vi "FPGA_Main_triple_SCTL.vi"() -> ()   [LabVIEW 2018]
uses:
  param-sctl-pll.ctl
  param-sctl-lockin.ctl
  scan param.ctl
  shutter-modes.ctl
  states.ctl
  <vilib>/Platform/TimedLoop/XDataNode/timing_clust.ctl
  <vilib>/Platform/TimedLoop/XDataNode/nitl_modes.ctl
  <vilib>/Platform/TimedLoop/XDataNode/wakeup.ctl
  <vilib>/rvi/Emulation/niFpgaGetClockAttributes.vi
  <vilib>/rvi/Emulation/niFpgaSctlEmulationGetInTimedLoop.vi
  <vilib>/rvi/Emulation/niFpgaEmulationReportErrorSimple.vi
  <vilib>/rvi/eio/common/nirviEmuTemplatePropertySet_noerrors.vi
  <vilib>/rvi/Emulation/niFpgaCriticalErrorInLSC.vi
  <vilib>/rvi/Emulation/niFpgaEmulationIsFPGAContextNoSignature.vi
  <vilib>/rvi/errors/niFpgaSetErrorForExecOnDevCompSimple.vi
  <vilib>/rvi/eio/common/nirviEmuReportErrorAndStop.vi
  <vilib>/rvi/DataTransferAndStorage/Container/Common/niFpgaContainerGetUniqueNameForEmu.vi
  <vilib>/rvi/FIFO/Fifo_Resource/nirvififoEmulationSetSize.vi
  <vilib>/rvi/FIFO/Fifo_Resource/nirviFifoEmulationQueueMgr.vi
  <instcachedir>/0/nirviFifoEmulationQueueMgr_E5CAEC123FF24DC58D834DCA3CDAA9B5.lvgen/nirviFifoEmulationQueueMgr_E5CAEC123FF24DC58D834DCA3CDAA9B5_000.vi
  <vilib>/Utility/error.llb/Clear Errors.vi
  <vilib>/rvi/FIFO/Fifo_Resource/nirvififoEmulationCreateLock.vi
  <vilib>/rvi/Emulation/niFpgaProcessEmulError.vi
  <vilib>/rvi/FIFO/Fifo_Resource/nirvififoEmulationObtainLock.vi
  <vilib>/rvi/FIFO/Fifo_Resource/nirvififoEmulationReleaseLock.vi
  <vilib>/rvi/occurrence/nirviWaitOnOccurrenceBase.vi
  <vilib>/rvi/errors/nirviReportUnexpectedCaseInternalError.vi
  <vilib>/rvi/errors/nirviReportUnexpectedCaseInternalError (U32).vi
  <vilib>/rvi/interface/RandomDataEmulation/niFpgaRandomDataHandleErrors.vi
  <vilib>/rvi/eio/common/nirviEmuTemplateMethod_errors.vi
  <vilib>/eio/EIOPropertyNode/EIOPropertyNode.xnode
  <vilib>/rvi/DataTransferAndStorage/Container/XNode/niFpgaContainer.xnode
  <vilib>/rvi/FIFO/Fifo_Resource/nirvififoEmulationRead.vi
  <vilib>/rvi/interface/RandomDataEmulation/nirviRandomDataFpgaReadWriteTemplate.vi
  <vilib>/eio/EIONode/EIONode.xnode
  <vilib>/Platform/TimedLoop/XDataNode/XDataNode.xnode
  <vilib>/rvi/DataTransferAndStorage/Handshake/Emulation/niFpgaHandshakeEmulation.vi
  <vilib>/rvi/eio/common/nirviEmuTemplatePropertyGet_errors.vi
  <vilib>/rvi/eio/common/nirviEmuTemplatePropertyGet_noerrors.vi
  <vilib>/rvi/eio/common/nirviEmuTemplatePropertySet_errors.vi
  PLL.lvlib
  SCTL.lvlib
  <vilib>/Platform/TimedLoop/XDataNode/XDNodeRunTimeDep.lvlib
  trigger-out.lvlib
  state machine.lvlib
panel:
  in  "enable BG log":bool
  out "APDs 2":u32[](array[numeric])
  out "x-y":u32[](array[numeric])
  out "APDs":u32[](array[numeric])
  in  "states":T1
  in  "stop":bool
  out "APDs pre-pixel":u32[](array[numeric])
  out "pixel counter":i16
  in  "line go!":bool
  out "curr state":T1
  in  "scan param":T2 {"pixel integration time (us)" format="%.2p"; "wait smaract (us)" format="%.2p"}
  out "Diode-in":fxp<+/-,27,5>
  in  "decimate":u8=1
  in  "analogue in settings":T4={"gain ch1"=1.0, "Voltage Range ch1"=enum."+/- 10 V", "gain ch2"=1.0, "Voltage Range ch1 2"=enum."+/- 10 V"}
  out "magnitude out":fxp<+,16,1>[](array[numeric])
  out "phases out":fxp<+,26,12>[](array[numeric])
  in  "param Lockin":T5={"harmonic"=[63.99993896484375, 63.99993896484375, 63.99993896484375], "LP1 coeffs"=[-1025014616, 2098093632, 165702, -1053286467, 2126356551, 167935, -1025014616, 2098093632, 165702, -1053286467, 2126356551, 167935, -1025014616, 2098093632, 165702, -1053286467, 2126356551, 167935], "scope on"=FALSE, "scope channel"=0, "scope signal"=0}
  in  "param PLL2":T6={"base freq (Hz)"=[20123.0, 20123.0, 20123.0], "P gain"=[1234.0, 1234.0, 1234.0], "I gain"=[1.0, 1.0, 1.0], "LP1 coeffs"=[-1025014616, 2098093632, 165702, -1053286467, 2126356551, 167935, -1025014616, 2098093632, 165702, -1053286467, 2126356551, 167935, -1025014616, 2098093632, 165702, -1053286467, 2126356551, 167935], "scope on"=FALSE, "scope channel"=0, "scope signal"=0, "notch coeff"=[-1025014616, 2098093632, 165702, -1053286467, 2126356551, 167935, -1025014616, 2098093632, 165702]}
  in  "param PLL1":T6={"base freq (Hz)"=[20123.0, 20123.0, 20123.0], "P gain"=[1234.0, 1234.0, 1234.0], "I gain"=[1.0, 1.0, 1.0], "LP1 coeffs"=[-1025014616, 2098093632, 165702, -1053286467, 2126356551, 167935, -1025014616, 2098093632, 165702, -1053286467, 2126356551, 167935, -1025014616, 2098093632, 165702, -1053286467, 2126356551, 167935], "scope on"=FALSE, "scope channel"=0, "scope signal"=0, "notch coeff"=[-1025014616, 2098093632, 165702, -1053286467, 2126356551, 167935, -1025014616, 2098093632, 165702]}
  out "phase error mean":fxp<+,16,1>[](array[numeric])
  out "freq error mean":fxp<+/-,16,11>[](array[numeric])
  in  "reset 3":bool
  out "AI data send at step #":i32=43
  in  "wait (clk)":u32=2 caption="wait"
  in  "idx  chan":u8
  out "timing wrong!":bool=TRUE
  out "loop time":u32=40
  in  "idx scope":u8=1
  in  "reset":bool
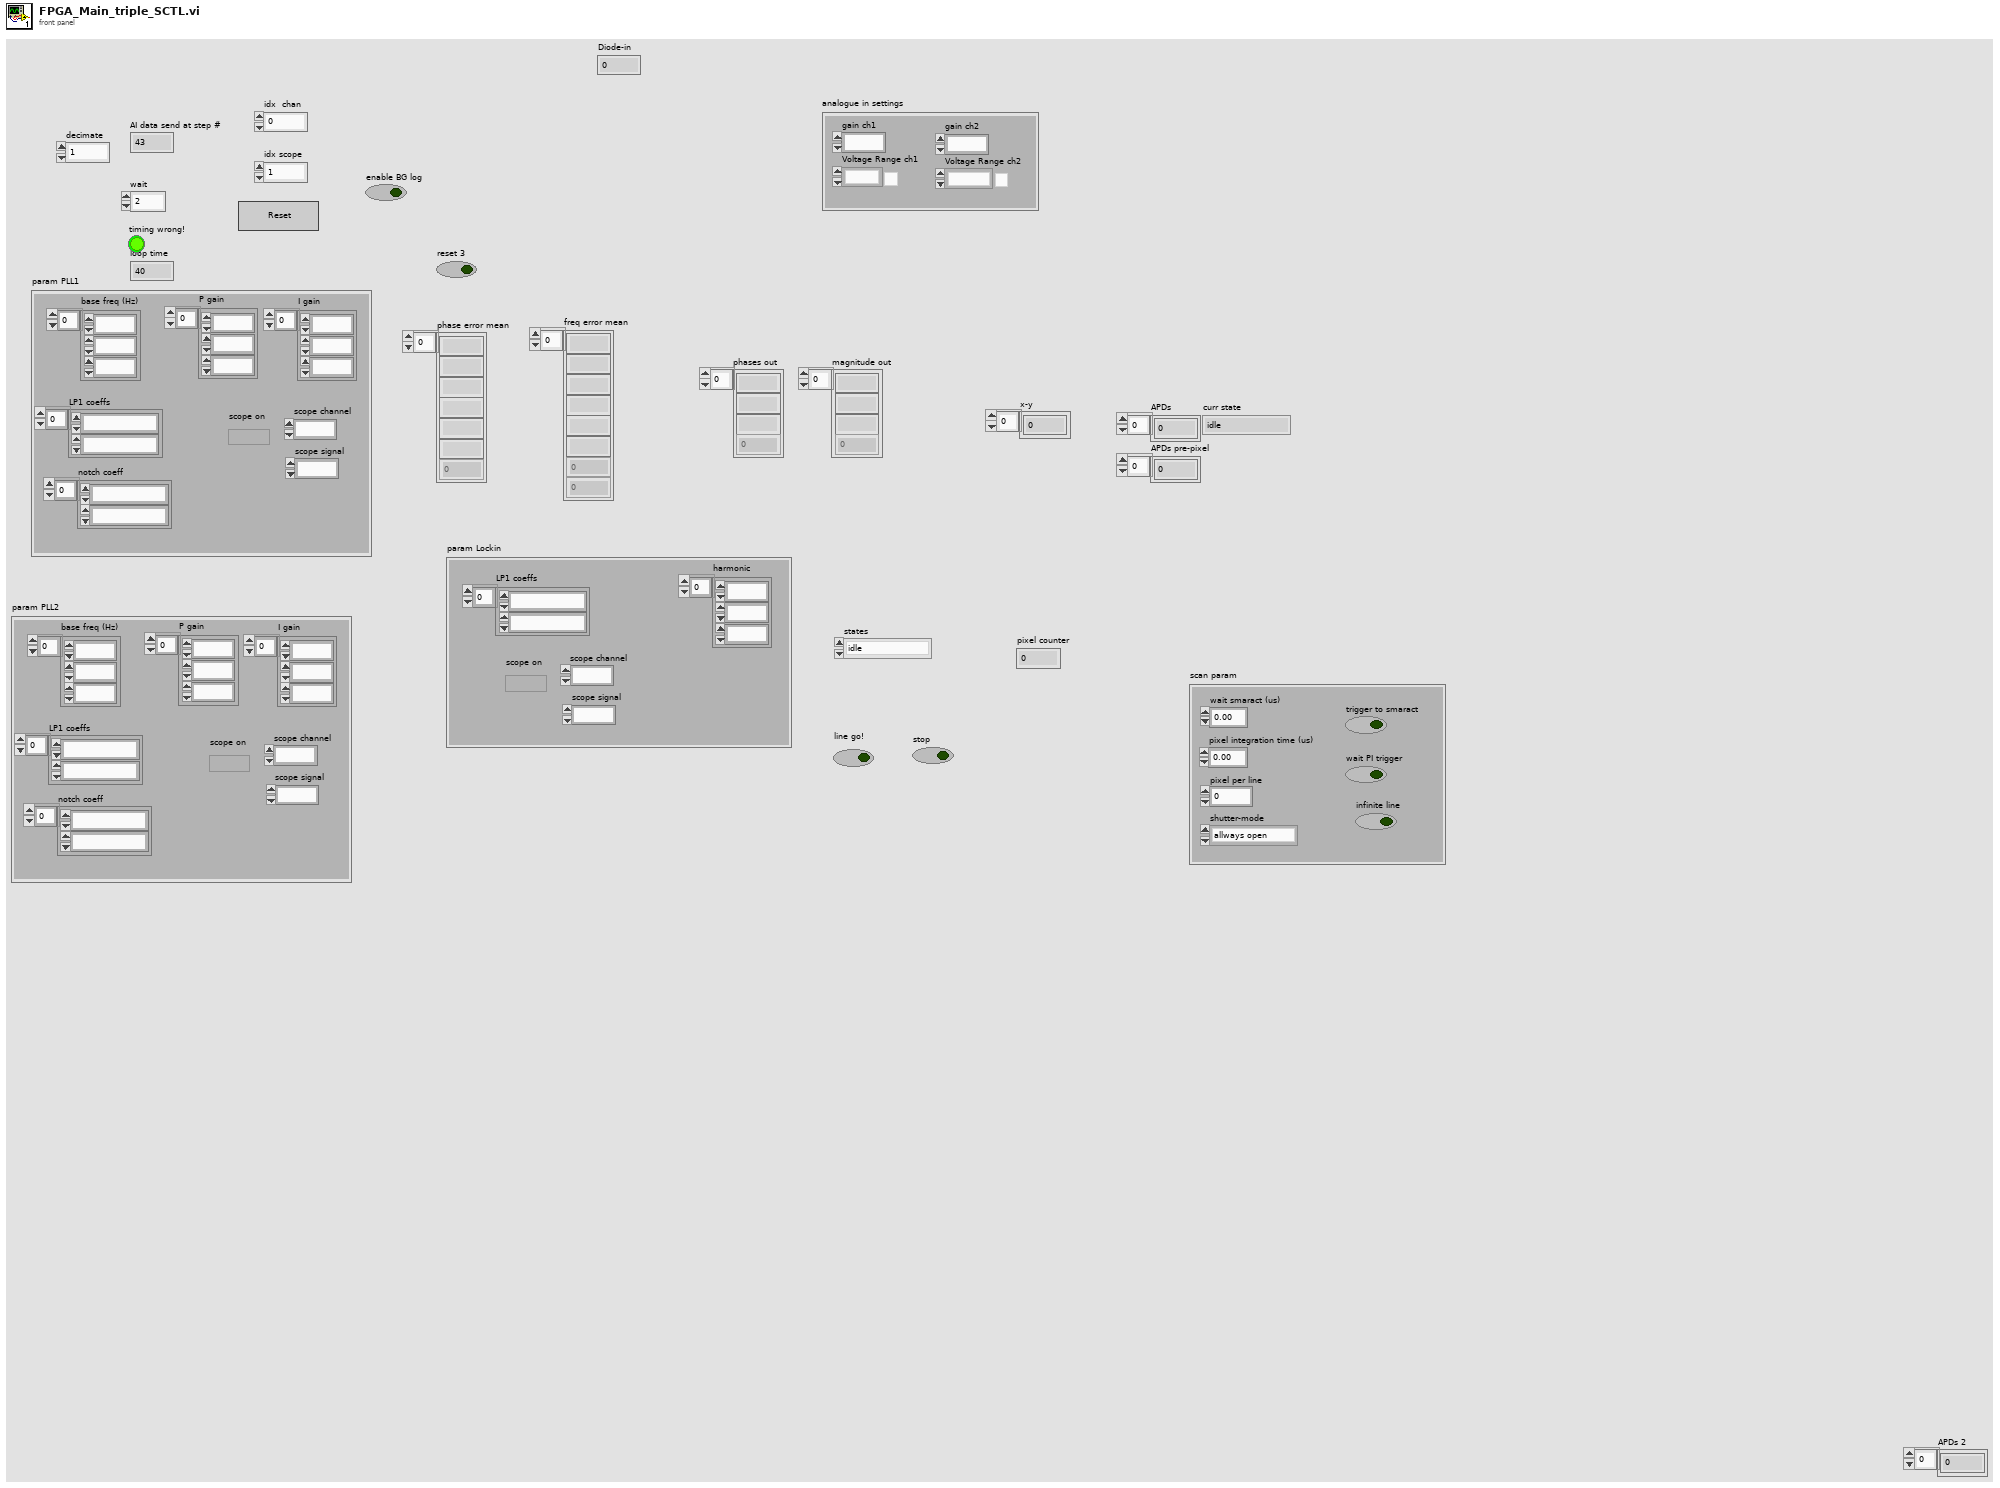
[diagram p1: front panel]
types:
  T1 = typedef "state machine.lvlib/states.ctl" = enum16{"idle", "pre-line", "pre-pixel", "pixel-integration", "pixel-readout", "post-pixel", "post-line"}
  T2 = typedef "state machine.lvlib/scan param.ctl" = cluster{"wait smaract (us)":u32, "pixel integration time (us)":u32, "pixel per line":i16, "shutter-mode":T3, "trigger to smaract":bool, "wait PI trigger":bool, "infinite line":bool}
  T3 = typedef "state machine.lvlib/shutter-modes.ctl" = enum16{"allways open", "allways closed", "open per line", "open per pixel"}
  T4 = cluster{"gain ch1":fxp<+,18,6>, "Voltage Range ch1":enum8{"+/- 10 V", "+/- 5 V", "+/- 2 V", "+/- 1 V"}, "gain ch2":fxp<+,18,6>, "Voltage Range ch1 2":enum8{"+/- 10 V", "+/- 5 V", "+/- 2 V", "+/- 1 V"}}
  T5 = typedef "param-sctl-lockin.ctl" = cluster{"harmonic":fxp<+,20,6>[], "LP1 coeffs":i32[], "scope on":bool, "scope channel":u8, "scope signal":u8}
  T6 = typedef "SCTL.lvlib/param-sctl-pll.ctl" = cluster{"base freq (Hz)":fxp<+,17,17>[], "P gain":fxp<+,14,14>[], "I gain":fxp<+,20,6>[], "LP1 coeffs":i32[], "scope on":bool, "scope channel":u8, "scope signal":u8, "notch coeff":i32[]}
  T7 = enum8{"+/- 10 V", "+/- 5 V", "+/- 2 V", "+/- 1 V"}
  T8 = typedef "XDNodeRunTimeDep.lvlib/timing_clust.ctl" = cluster{"Expected End [f-1]":u64, "Actual End [f-1]":u64, "Finished Late? [f-1]":bool, "Expected End [i-1]":u64, "Actual End [i-1]":u64, "Finished Late? [i-1]":bool, "Expected Start [i]":u64, "Actual Start [i]":u64, "Expected Start [f]":u64, "Actual Start [f]":u64, "Source Name":string, "Structure Name":string, "Period":i64, "Deadline":i64, "Offset":i64, "Start":i64, "Priority":i32, "Timeout":i32, "Mode":T9, "Wakeup Reason":T10, "Error":errorcluster, "Source Type":string, "Secondary Source Type":string, "Global End Time":u64, "Global Start Time":u64, "Frame Duration":u64, "Iteration Duration":u64, "Assigned CPU":i32, "I/O Scan Engine Mode":u32}
  T9 = typedef "XDNodeRunTimeDep.lvlib/nitl_modes.ctl" = enum32{"No Change", "Process missed periods, maintain original phase", "Discard missed periods, maintain original phase", "Process missed periods, ignore original phase", "Discard missed periods, ignore original phase"}
  T10 = typedef "XDNodeRunTimeDep.lvlib/wakeup.ctl" = enum32{"Normal", "Aborted", "Asynchronous wakeup", "Timing source error", "Timed loop error", "Timeout"}
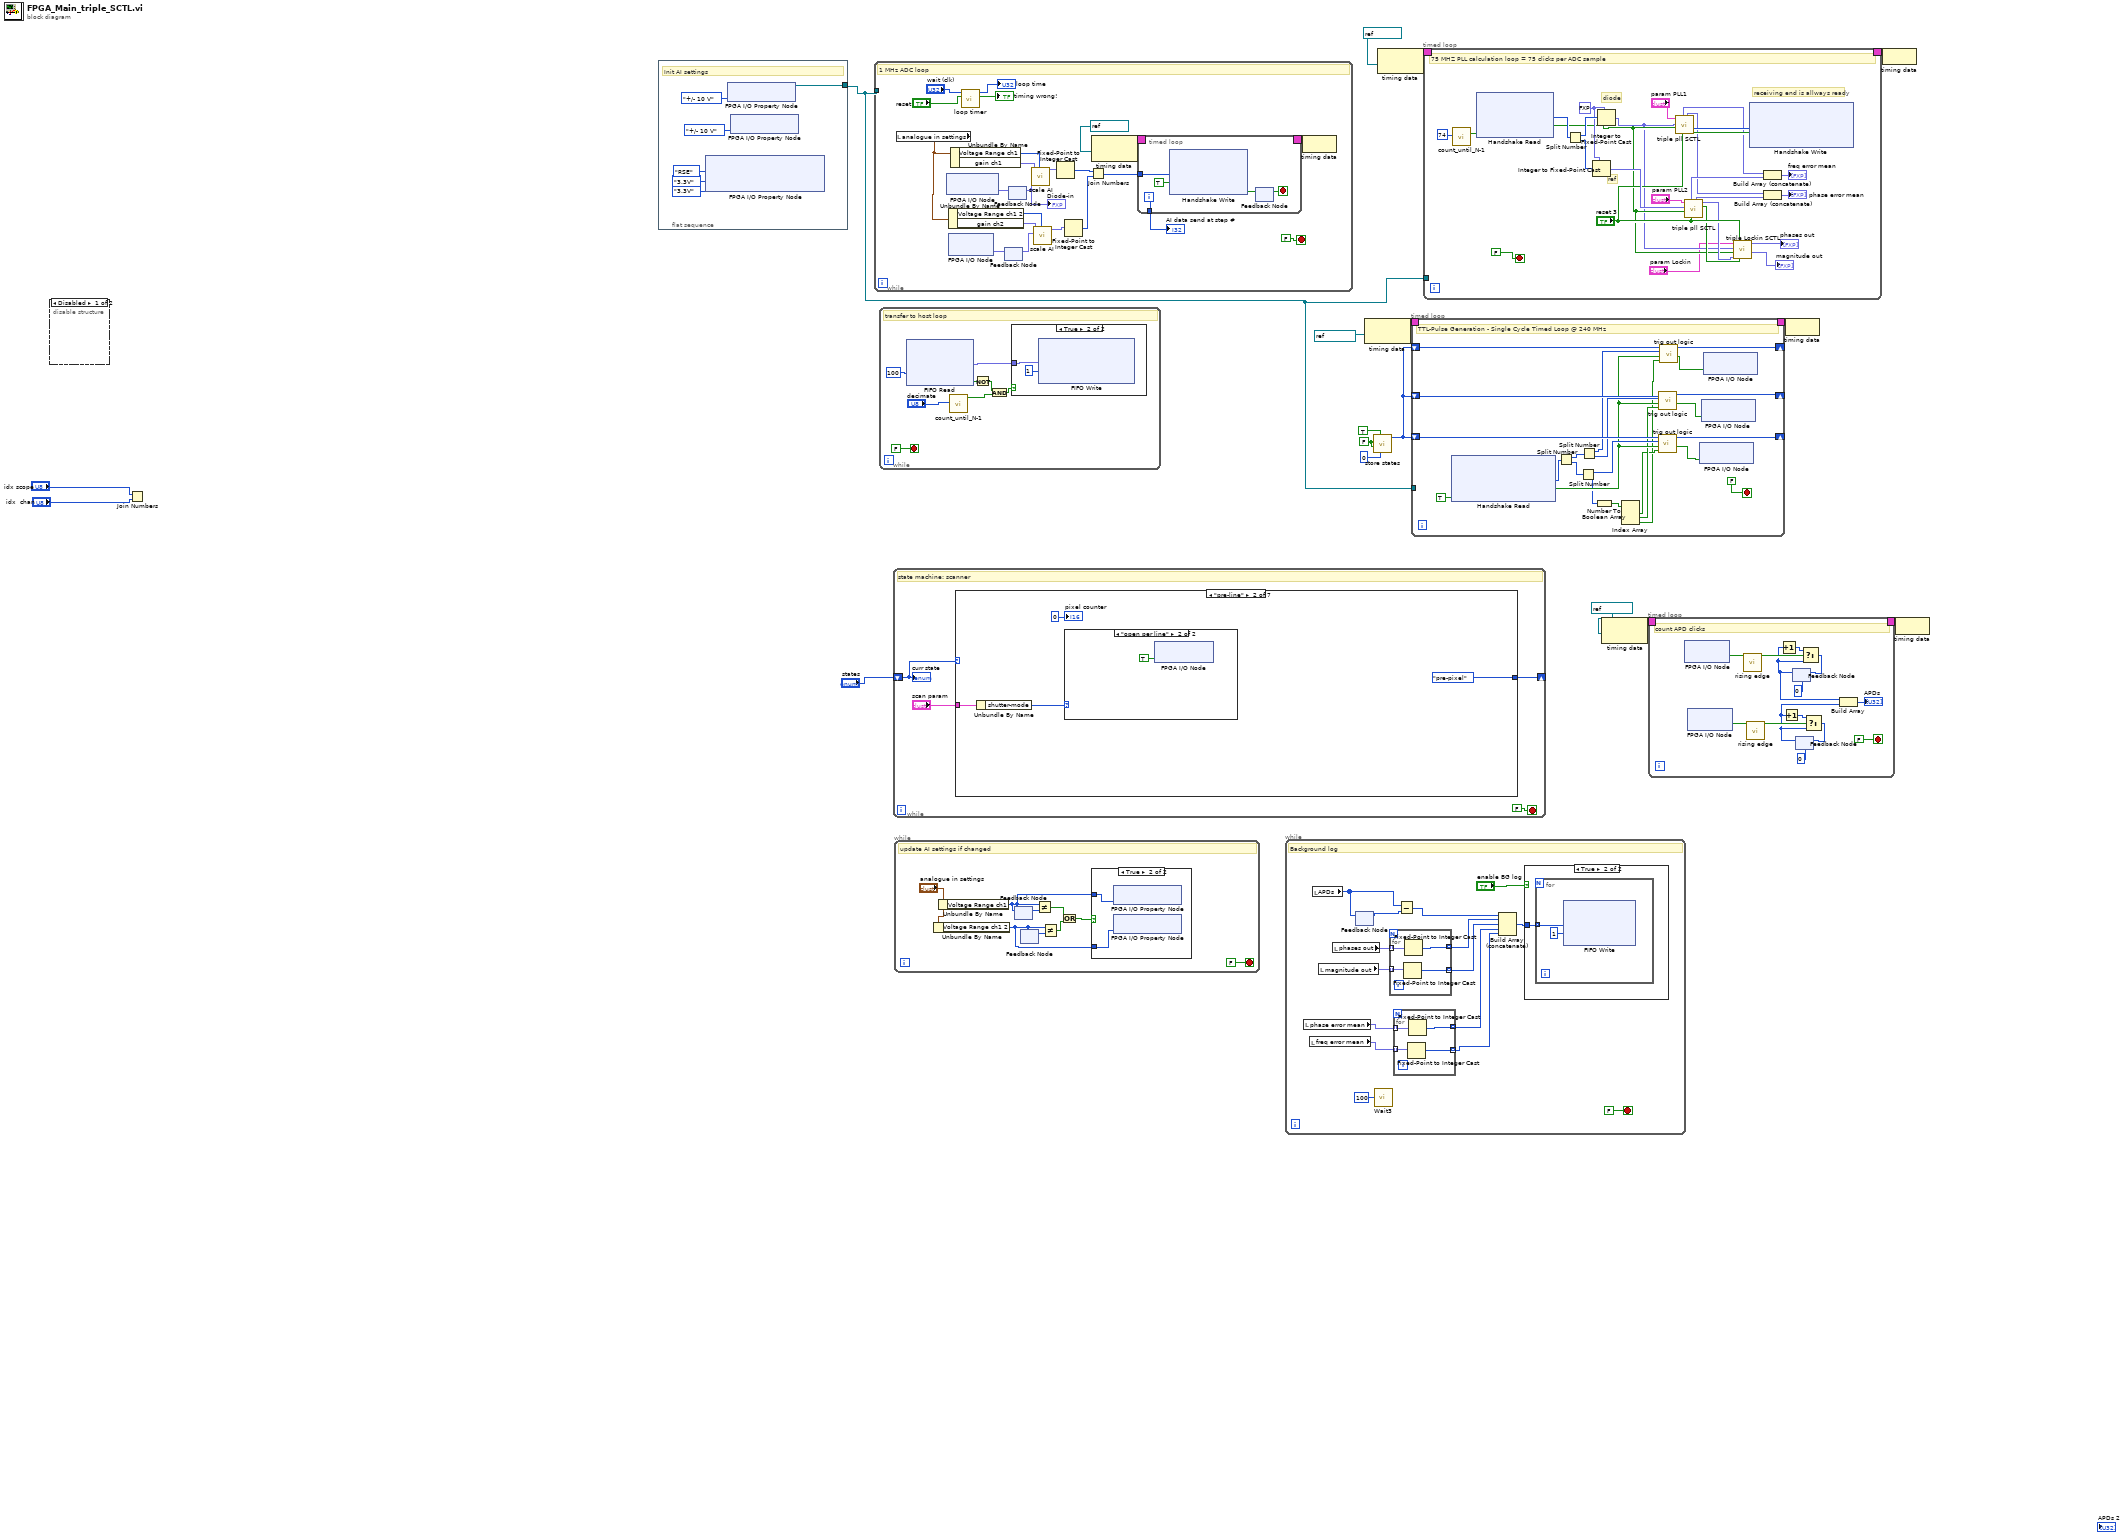
[diagram p0: block diagram]
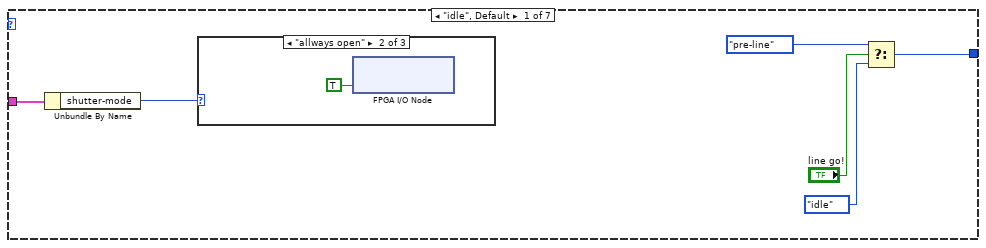
[diagram p5: hidden frame]
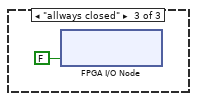
[diagram p7: hidden frame]
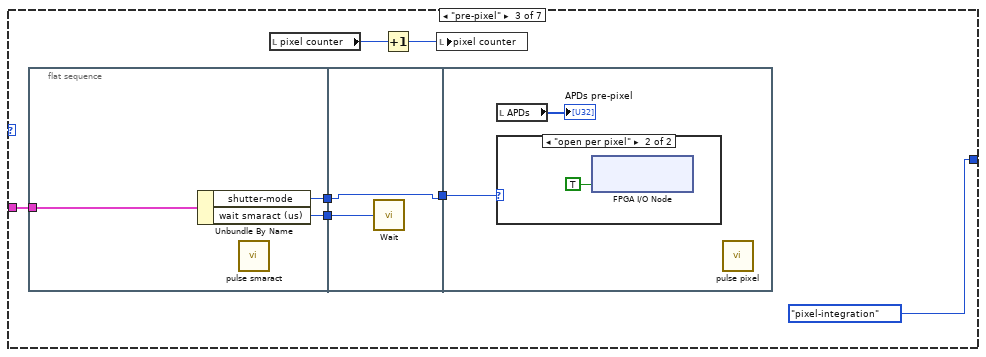
[diagram p9: hidden frame]
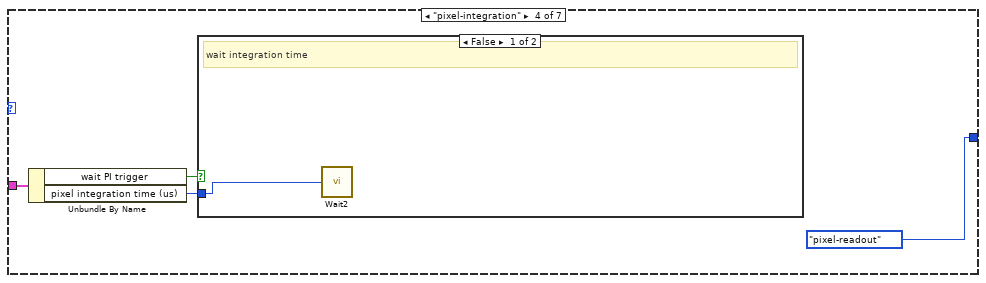
[diagram p11: hidden frame]
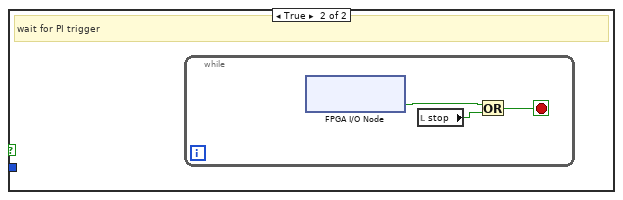
[diagram p12: hidden frame]
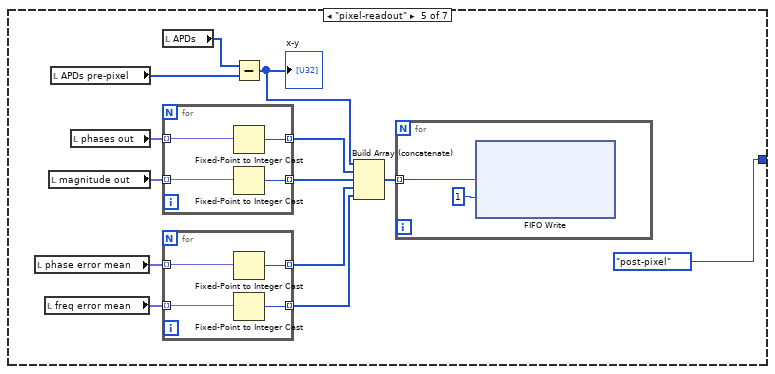
[diagram p13: hidden frame]
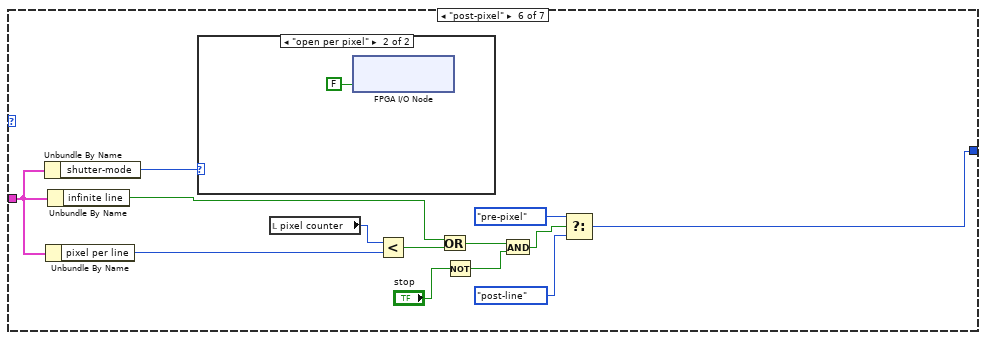
[diagram p14: hidden frame]
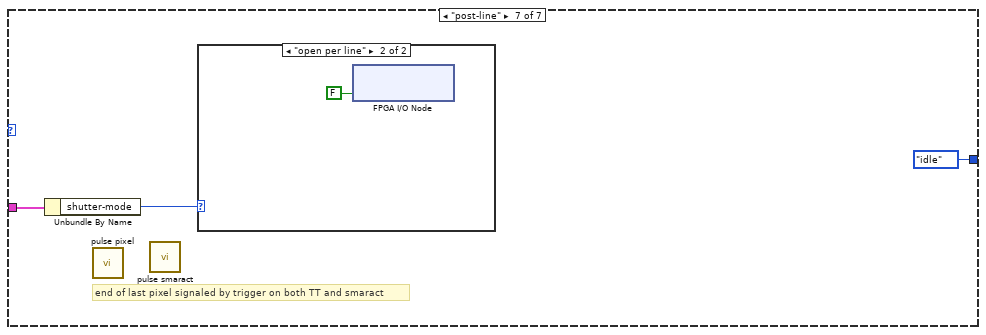
[diagram p16: hidden frame]
diagram:
  w4 = FALSE ("current output")
  n1 = disable-structure shown="Disabled" {
    frame Disabled {
    }
    frame Enabled {
    }
  }
  n2 = Join Numbers(hi="idx scope", lo="idx  chan") -> ()  [unwired: 1 out]
  n3 = flat-sequence {
    tunnel: [w20] -> w1
    frame #0 {
      # "Init AI settings"
      n4 = xnode "FPGA I/O Property Node"("AI Terminal Mode"=enum8{"DIFF", "RSE", "NRSE"}."RSE", "Connector1:2 DIO Logic Family"=enum8{"3.3V", "2.5V", "1.8V", "1.5V", "1.2V"}."3.3V", "Connector3 DIO Logic Family"=enum8{"3.3V", "2.5V", "1.8V", "1.5V", "1.2V"}."3.3V") -> ()  [unwired: 1 in, 1 out]
      n5 = xnode "FPGA I/O Property Node"("Voltage Range"=T7."+/- 10 V") -> ("FPGA I/O Out"=w20:refnum<k21>)  [unwired: 1 in]
      n6 = xnode "FPGA I/O Property Node"("Voltage Range"=T7."+/- 10 V") -> ()  [unwired: 1 in, 1 out]
    }
  }
  n7 = while {
    tunnel: w1 -> [_]
    stop <- FALSE stop-if-true
    # "1 MHz ADC loop"
    n8 = local read "analogue in settings"() -> (w27:T4)
    n9 = xnode "FPGA I/O Node"() -> ("Diode-in"=w42:fxp<+/-,27,5>)  [unwired: 1 in, 1 out]
    n10 = Unbundle By Name(w27) -> ("Voltage Range ch1 2"=w24:T7, "gain ch2"=w26:fxp<+,18,6>)
    n11 = xnode "FPGA I/O Node"() -> ("Ref-in"=w34:fxp<+/-,27,5>)  [unwired: 1 in, 1 out]
    n12 = Unbundle By Name(w27) -> ("Voltage Range ch1"=w25:T7, "gain ch1"=w28:fxp<+,18,6>)
    n13 = call "loop timer.vi"("reset"="reset", "wait"="wait (clk)") -> ("timing wrong"=→"timing wrong!":bool, "loop time out"=→"loop time":u32)  [unwired: 8 in]
    n14 = feedback #1() -> (w35:fxp<+/-,27,5>)  [unwired: 1 in]
    n15 = feedback-in #1(w34) -> ()
    n16 = feedback #2() -> (w41:fxp<+/-,27,5>)  [unwired: 1 in]
    "Diode-in" <- w41
    n17 = feedback-in #2(w42) -> ()
    n18 = call "scale AI.vi"("Voltage Range ch2"=w25, "Ref-In"=w41, "gain"=w28) -> ("signal"=w30:fxp<+/-,17,1>)  [unwired: 8 in]
    n19 = call "scale AI.vi"("Voltage Range ch2"=w24, "Ref-In"=w35, "gain"=w26) -> ("signal"=w33:fxp<+/-,17,1>)  [unwired: 8 in]
    n20 = Fixed-Point to Integer Cast(1:w30) -> (0:w32:i32)
    n21 = Fixed-Point to Integer Cast(1:w33) -> (0:w31:i32)
    n22 = Join Numbers(hi=w32, lo=w31) -> ((hi.lo)=w29:u64)
    n23 = node-c288(refnum<k21> "75MHz" ("Source Name")) -> (w45:T8)
    n24 = timed-loop {
      timing: w45 -> [_]
      timing-out: [_] -> w44
      tunnel: w29 -> [w51]
      tunnel: [w49] -> w36
      i -> [w49]
      stop <- w47 stop-if-true
      n25 = xnode ("Handshake Write")("Data"=w51, "Input Valid"=TRUE) -> ("Ready for Input"=w48:bool)  [unwired: 1 in, 1 out]
      n26 = feedback-in #3(w48) -> ()
      n27 = feedback #3() -> (w47:bool)  [unwired: 1 in]
    }
    "AI data send at step #" <- w36
    n28 = node-c288(w44) -> ()
  }
  n29 = while {
    stop <- FALSE stop-if-true
    # "transfer to host loop"
    n30 = xnode ("FIFO Read")("Timeout"=100) -> ("Element"=w64:fxp<+/-,16,1>, "Timed Out?"=w62:bool)  [unwired: 1 in, 1 out]
    n31 = call "count_until_N-1.vi"("N"="decimate") -> ("turn around !"=w59:bool)  [unwired: 9 in, 1 out]
    n32 = Not(x=w62) -> (.not. x?=w61:bool)
    n33 = And(x=w61, y=w59) -> (x .and. y?=w60:bool)
    n34 = case shown="True" w60 {
      tunnel: w64 -> [_ w67]
      frame False {
      }
      frame True {
        n35 = xnode ("FIFO Write")("Element"=w67, "Timeout"=i16 1 ("Numeric")) -> ()  [unwired: 1 in, 2 out]
      }
    }
  }
  n36 = while {
    shift-right: [w70] -> _
    shift-left: "states" -> [w69]
    stop <- FALSE stop-if-true
    # "state machine: scanner"
    n37 = case shown="\"pre-line\"" w69 {
      tunnel: [w76 states."pre-pixel" ("states") states."pixel-integration" ("states") states."pixel-readout" ("states") states."post-pixel" ("states") w139 states."idle" ("states")] -> w70
      tunnel: "scan param" -> [w72 w80 w88 w102 _ w134 w145]
      frame "idle", Default {
        n38 = Unbundle By Name(w72) -> ("shutter-mode"=w73:T3)
        n39 = case shown="\"allways open\"" w73 {
          frame "open per line", Default {
          }
          frame "allways open" {
            n40 = xnode "FPGA I/O Node"("shutter out"=TRUE) -> ()  [unwired: 1 in, 1 out]
          }
          frame "allways closed" {
            n41 = xnode "FPGA I/O Node"("shutter out"=FALSE) -> ()  [unwired: 1 in, 1 out]
          }
        }
        n42 = Select(t=states."pre-line" ("states"), s="line go!", f=states."idle" ("states")) -> (s? t:f=w76:T1)
      }
      frame "pre-line" {
        n43 = Unbundle By Name(w80) -> ("shutter-mode"=w81:T3)
        n44 = case shown="\"open per line\"" w81 {
          frame "allways open", Default {
          }
          frame "open per line" {
            n45 = xnode "FPGA I/O Node"("shutter out"=TRUE) -> ()  [unwired: 1 in, 1 out]
          }
        }
        "pixel counter" <- i16 0 ("pixel counter")
      }
      frame "pre-pixel" {
        n46 = flat-sequence {
          tunnel: [w94] -> w87
          tunnel: w88 -> [w93]
          tunnel: [w92] -> w85
          tunnel: w87 -> [w96]
          tunnel: [w96] -> w86
          tunnel: w85 -> [w95]
          tunnel: w86 -> [w97]
          frame #0 {
            n47 = Unbundle By Name(w93) -> ("shutter-mode"=w94:T3, "wait smaract (us)"=w92:u32)
            n48 = call "pulse smaract.vi"() -> ()  [unwired: 12 in]
          }
          frame #1 {
            n49 = call "Wait"("Count(uSec)"=w95) -> ()  [unwired: 1 out]
          }
          frame #2 {
            n50 = local read "APDs"() -> (→"APDs pre-pixel":u32[])
            n51 = case shown="\"open per pixel\"" w97 {
              frame "allways open", Default {
              }
              frame "open per pixel" {
                n52 = xnode "FPGA I/O Node"("shutter out"=TRUE) -> ()  [unwired: 1 in, 1 out]
              }
            }
            n53 = call "pulse pixel.vi"() -> ()  [unwired: 12 in]
          }
        }
        n54 = local read "pixel counter"() -> (w91:i16)
        n55 = Increment(x=w91) -> (x+1=w90:i16)
        n56 = local write "pixel counter"(w90) -> ()
      }
      frame "pixel-integration" {
        n57 = Unbundle By Name(w102) -> ("wait PI trigger"=w101:bool, "pixel integration time (us)"=w100:u32)
        n58 = case shown="False" w101 {
          tunnel: w100 -> [w104 _]
          frame False {
            # "wait integration time"
            n59 = call "Wait2"("Count(uSec)"=w104) -> ()  [unwired: 1 out]
          }
          frame True {
            # "wait for PI trigger"
            n60 = while {
              stop <- w107 stop-if-true
              n61 = xnode "FPGA I/O Node"() -> ("PI stage IN"=w106:bool)  [unwired: 1 in, 1 out]
              n62 = local read "stop"() -> (w105:bool)
              n63 = Or(x=w106, y=w105) -> (x .or. y?=w107:bool)
            }
          }
        }
      }
      frame "pixel-readout" {
        n64 = local read "phase error mean"() -> (w115:fxp<+,16,1>[])
        n65 = local read "freq error mean"() -> (w114:fxp<+/-,16,11>[])
        n66 = local read "magnitude out"() -> (w116:fxp<+,16,1>[])
        n67 = local read "APDs pre-pixel"() -> (w118:u32[])
        n68 = local read "phases out"() -> (w117:fxp<+,26,12>[])
        n69 = local read "APDs"() -> (w119:u32[])
        n70 = for {
          tunnel: w117 -> [w130] mode=indexing
          tunnel: [w129] -> w112 mode=indexing
          tunnel: w116 -> [w128] mode=indexing
          tunnel: [w127] -> w111 mode=indexing
          n71 = Fixed-Point to Integer Cast(1:w130) -> (0:w129:u32)
          n72 = Fixed-Point to Integer Cast(1:w128) -> (0:w127:u16)
        }
        n73 = for {
          tunnel: w115 -> [w126] mode=indexing
          tunnel: [w125] -> w110 mode=indexing
          tunnel: w114 -> [w124] mode=indexing
          tunnel: [w123] -> w109 mode=indexing
          n74 = Fixed-Point to Integer Cast(1:w126) -> (0:w125:u16)
          n75 = Fixed-Point to Integer Cast(1:w124) -> (0:w123:i16)
        }
        n76 = Subtract(x=w119, y=w118) -> (x-y=w113:u32[])
        "x-y" <- w113
        n77 = Build Array (concatenate)(w113, w112, w111, w110, w109) -> (w108:u32[])
        n78 = for {
          tunnel: w108 -> [w122] mode=indexing
          n79 = xnode ("FIFO Write")("Element"=w122, "Timeout"=1) -> ()  [unwired: 1 in, 2 out]
        }
      }
      frame "post-pixel" {
        n80 = Unbundle By Name(w134) -> ("shutter-mode"=w136:T3)
        n81 = Unbundle By Name(w134) -> ("pixel per line"=w135:i16)
        n82 = Unbundle By Name(w134) -> ("infinite line"=w133:bool)
        n83 = case shown="\"open per pixel\"" w136 {
          frame "allways open", Default {
          }
          frame "open per pixel" {
            n84 = xnode "FPGA I/O Node"("shutter out"=FALSE) -> ()  [unwired: 1 in, 1 out]
          }
        }
        n85 = local read "pixel counter"() -> (w143:i16)
        n86 = Less?(x=w143, y=w135) -> (x < y?=w132:bool)
        n87 = Or(x=w133, y=w132) -> (x .or. y?=w131:bool)
        n88 = Not(x="stop") -> (.not. x?=w141:bool)
        n89 = And(x=w131, y=w141) -> (x .and. y?=w140:bool)
        n90 = Select(t=states."pre-pixel" ("states"), s=w140, f=states."post-line" ("states")) -> (s? t:f=w139:T1)
      }
      frame "post-line" {
        # "end of last pixel signaled by trigger on both TT and smaract"
        n91 = Unbundle By Name(w145) -> ("shutter-mode"=w146:T3)
        n92 = call "pulse pixel.vi"() -> ()  [unwired: 12 in]
        n93 = call "pulse smaract.vi"() -> ()  [unwired: 12 in]
        n94 = case shown="\"open per line\"" w146 {
          frame "allways open", Default {
          }
          frame "open per line" {
            n95 = xnode "FPGA I/O Node"("shutter out"=FALSE) -> ()  [unwired: 1 in, 1 out]
          }
        }
      }
    }
    "curr state" <- w69
  }
  n96 = while {
    stop <- FALSE stop-if-true
    # "update AI settings if changed"
    n97 = Unbundle By Name("analogue in settings") -> ("Voltage Range ch1 2"=w150:T7)
    n98 = Unbundle By Name("analogue in settings") -> ("Voltage Range ch1"=w151:T7)
    n99 = feedback-in #4(w151) -> ()
    n100 = feedback #4() -> (w157:T7)  [unwired: 1 in]
    n101 = feedback #5() -> (w155:T7)  [unwired: 1 in]
    n102 = feedback-in #5(w150) -> ()
    n103 = Not Equal?(x=w151, y=w157) -> (x != y?=w153:bool)
    n104 = Not Equal?(x=w150, y=w155) -> (x != y?=w154:bool)
    n105 = Or(x=w153, y=w154) -> (x .or. y?=w152:bool)
    n106 = case shown="True" w152 {
      tunnel: w151 -> [_ w159]
      tunnel: w150 -> [_ w158]
      frame False {
      }
      frame True {
        n107 = xnode "FPGA I/O Property Node"("Voltage Range"=w159) -> ()  [unwired: 1 in, 1 out]
        n108 = xnode "FPGA I/O Property Node"("Voltage Range"=w158) -> ()  [unwired: 1 in, 1 out]
      }
    }
  }
  n109 = while {
    stop <- FALSE stop-if-true
    # "Background log"
    n110 = local read "phase error mean"() -> (w172:fxp<+,16,1>[])
    n111 = local read "freq error mean"() -> (w171:fxp<+/-,16,11>[])
    n112 = local read "APDs"() -> (w164:u32[])
    n113 = local read "magnitude out"() -> (w173:fxp<+,16,1>[])
    n114 = local read "phases out"() -> (w174:fxp<+,26,12>[])
    n115 = feedback-in #6(w164) -> ()
    n116 = feedback #6() -> (w163:u32[])  [unwired: 1 in]
    n117 = call "Wait3"("Count(mSec)"=u32 100) -> ()  [unwired: 1 out]
    n118 = for {
      tunnel: w174 -> [w185] mode=indexing
      tunnel: [w184] -> w169 mode=indexing
      tunnel: w173 -> [w183] mode=indexing
      tunnel: [w182] -> w168 mode=indexing
      n119 = Fixed-Point to Integer Cast(1:w183) -> (0:w182:u16)
      n120 = Fixed-Point to Integer Cast(1:w185) -> (0:w184:u32)
    }
    n121 = for {
      tunnel: w172 -> [w181] mode=indexing
      tunnel: [w180] -> w167 mode=indexing
      tunnel: w171 -> [w179] mode=indexing
      tunnel: [w178] -> w166 mode=indexing
      n122 = Fixed-Point to Integer Cast(1:w179) -> (0:w178:i16)
      n123 = Fixed-Point to Integer Cast(1:w181) -> (0:w180:u16)
    }
    n124 = Subtract(x=w164, y=w163) -> (x-y=w170:u32[])
    n125 = Build Array (concatenate)(w170, w169, w168, w167, w166) -> (w165:u32[])
    n126 = case shown="True" "enable BG log" {
      tunnel: w165 -> [_ w175]
      frame False {
      }
      frame True {
        n127 = for {
          tunnel: w175 -> [w177] mode=indexing
          n128 = xnode ("FIFO Write")("Element"=w177, "Timeout"=1) -> ()  [unwired: 1 in, 2 out]
        }
      }
    }
  }
  n129 = node-c288(refnum<k21> "240MHz" ("Source Name")) -> (w9:T8)
  n130 = call "store states.vi"("counter index"=u8 0, "pulse not yet sent"=TRUE, "next output"=w4, "current output"=w4) -> ("state out"=w6:u16)  [unwired: 7 in]
  n131 = node-c288(refnum<k21> "75MHz" ("Source Name")) -> (w11:T8)
  n132 = timed-loop {
    timing: w9 -> [_]
    timing-out: [_] -> w8
    shift-right: [w205] -> _
    shift-left: w6 -> [w206]
    shift-right: [w198] -> _
    shift-left: w6 -> [w201]
    shift-right: [w199] -> _
    shift-left: w6 -> [w200]
    tunnel: w1 -> [_]
    stop <- FALSE stop-if-true
    # "TTL-Pulse Generation - Single Cycle Timed Loop @ 240 MHz"
    n133 = xnode ("Handshake Read")("Ready for Output"=TRUE) -> ("Data"=w204:u32, "Output Valid"=w194:bool)  [unwired: 1 in, 1 out]
    n134 = Split Number(x=w204) -> (hi(x)=w203:u16, lo(x)=w202:u16)
    n135 = Split Number(x=w202) -> (hi(x)=w195:u8, lo(x)=w190:u8)
    n136 = Split Number(x=w203) -> (hi(x)=w197:u8, lo(x)=w196:u8)
    n137 = Number To Boolean Array(number=w190) -> (Boolean array=w189:bool[])
    n138 = Index Array(array=w189) -> (element #1=w187:bool, element #2=w188:bool, element #3=w186:bool)  [unwired: 3 in]
    n139 = call "trig out logic.vi"("rising edge"=w187, "Output Valid"=w194, "pulse idx"=w195, "state in"=w206) -> ("output"=w191:bool, "state out out"=w205:u16)  [unwired: 6 in]
    n140 = call "trig out logic.vi"("rising edge"=w188, "Output Valid"=w194, "pulse idx"=w196, "state in"=w201) -> ("output"=w192:bool, "state out out"=w198:u16)  [unwired: 6 in]
    n141 = call "trig out logic.vi"("rising edge"=w186, "Output Valid"=w194, "pulse idx"=w197, "state in"=w200) -> ("output"=w193:bool, "state out out"=w199:u16)  [unwired: 6 in]
    n142 = xnode "FPGA I/O Node"("TTL-out1"=w191) -> ()  [unwired: 1 in, 1 out]
    n143 = xnode "FPGA I/O Node"("TTL-out2"=w192) -> ()  [unwired: 1 in, 1 out]
    n144 = xnode "FPGA I/O Node"("TTL-out3"=w193) -> ()  [unwired: 1 in, 1 out]
  }
  n145 = timed-loop "Timed Loop" {
    timing: w11 -> [_]
    timing-out: [_] -> w10
    tunnel: w1 -> [_]
    stop <- FALSE stop-if-true
    w221 = fxp<+/-,17,1> 0.0 ("fixed-point")
    # "receiving end is allways ready"
    # "ref"
    # "diode"
    # "75 MHZ PLL calculation loop = 75 clicks per ADC sample"
    n146 = call "count_until_N-1.vi"("N"=u8 74) -> ("turn around !"=w235:bool)  [unwired: 9 in, 1 out]
    n147 = xnode ("Handshake Read")("Ready for Output"=w235) -> ("Data"=w224:u64, "Output Valid"=w216:bool)  [unwired: 1 in, 1 out]
    n148 = Split Number(x=w224) -> (hi(x)=w223:u32, lo(x)=w222:u32)
    n149 = Integer to Fixed-Point Cast(fixed-point type=w221, integer=w222) -> (fixed-point=w220:fxp<+/-,17,1>)
    n150 = Integer to Fixed-Point Cast(fixed-point type=w221, integer=w223) -> (fixed-point=w215:fxp<+/-,17,1>)
    n151 = call "triple pll SCTL.vi"("reset"="reset 3", "AI Valid"=w216, "AI in"=w215, "param"="param PLL1") -> ("pulse valid"=w233:bool, "3 pulse idx"=w234:u32, "phase errror mean out"=w229:fxp<+,16,1>[], "freq error mean out"=w231:fxp<+/-,16,11>[])  [unwired: 1 in, 3 out]
    n152 = call "triple pll SCTL.vi"("reset"="reset 3", "AI Valid"=w216, "AI in"=w220, "param"="param PLL2") -> ("phase block valid"=w217:bool, "phases out"=w218:fxp<+,26,1>[], "phase errror mean out"=w228:fxp<+,16,1>[], "freq error mean out"=w232:fxp<+/-,16,11>[])  [unwired: 1 in, 3 out]
    n153 = call "triple Lockin SCTL.vi"("phases valid"=w217, "reset"="reset 3", "phases in"=w218, "AI Valid"=w216, "AI in"=w215, "param"="param Lockin") -> ("magnitude out"=→"magnitude out":fxp<+,16,1>[], "unwrapped phases out"=→"phases out":fxp<+,26,12>[])  [unwired: 3 in, 1 out]
    n154 = xnode ("Handshake Write")("Data"=w234, "Input Valid"=w233) -> ()  [unwired: 1 in, 2 out]
    n155 = Build Array (concatenate)(w231, w232) -> (→"freq error mean":fxp<+/-,16,11>[])
    n156 = Build Array (concatenate)(w229, w228) -> (→"phase error mean":fxp<+,16,1>[])
  }
  n157 = node-c288(refnum<k21> "240MHz" ("Source Name")) -> (w14:T8)
  n158 = timed-loop {
    timing: w14 -> [_]
    timing-out: [_] -> w13
    stop <- FALSE stop-if-true
    # "count APD clicks"
    n159 = xnode "FPGA I/O Node"() -> ("APD1"=w251:bool)  [unwired: 1 in, 1 out]
    n160 = xnode "FPGA I/O Node"() -> ("APD2"=w247:bool)  [unwired: 1 in, 1 out]
    n161 = call "rising edge.vi"("APD1"=w251) -> ("Boolean"=w250:bool)  [unwired: 10 in]
    n162 = call "rising edge.vi"("APD1"=w247) -> ("Boolean"=w246:bool)  [unwired: 10 in]
    n163 = feedback #7(u32 0) -> (w241:u32)
    n164 = Increment(x=w241) -> (x+1=w249:u32)
    n165 = feedback #8(u32 0) -> (w240:u32)
    n166 = Increment(x=w240) -> (x+1=w245:u32)
    n167 = Select(t=w249, s=w250, f=w241) -> (s? t:f=w242:u32)
    n168 = feedback-in #7(w242) -> ()
    n169 = Select(t=w245, s=w246, f=w240) -> (s? t:f=w243:u32)
    n170 = feedback-in #8(w243) -> ()
    n171 = Build Array(w241, w240) -> (→"APDs":u32[])
  }
  n172 = node-c288(w8) -> ()
  n173 = node-c288(w10) -> ()
  n174 = node-c288(w13) -> ()
